vi "Inspect Tell.vi"(4 "Alias":string, 6 "Msg":refnum<class "Msg.lvclass">, 10 "Teller":T1 {"Absolute Time" format="%<%x %.3X>T"}, 11 "Base Actor in":refnum<class "Base Actor.lvclass">) -> (0 "Error out":errorcluster, 3 "Base Actor out":refnum<class "Base Actor.lvclass">)   [LabVIEW 2020, in "jettl.lvlib" / "Base jettl Actor.lvlib" / "Base Actor.lvlib" / "Base Actor.lvclass"]
uses:
  Base Actor.lvclass
  Base Actor.lvclass/Base Actor.ctl
  Relation.ctl
  jettl.lvlib
  Teller.ctl
  Msg/Msg.lvclass
  Transport/Transport.lvclass
  Actor/Actor.lvclass
  Msgs.ctl
  Unified Layer.ctl
  Actor Attributes.ctl
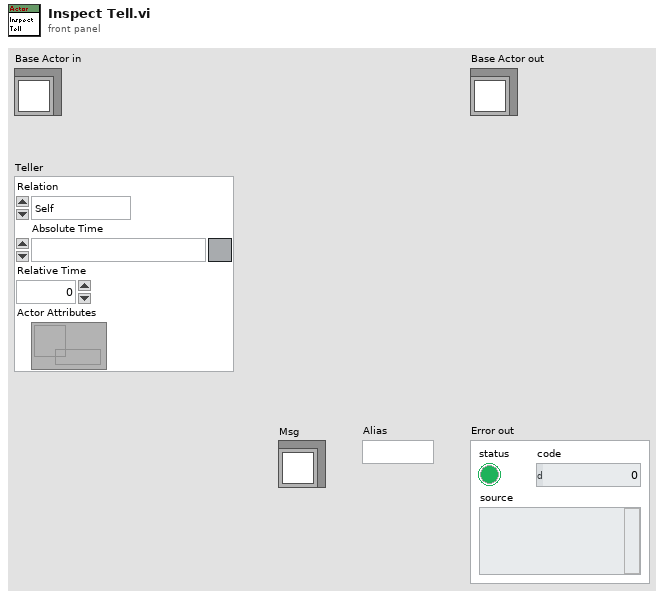
[diagram p1: front panel]
types:
  T1 = typedef "jettl.lvlib/Teller.ctl" = cluster{"Relation":T2, "Absolute Time":timestamp, "Relative Time":dbl, "Actor Attributes":refnum<data-value>}
  T2 = typedef "jettl.lvlib/Relation.ctl" = enum16{"Self", "Parent", "Child"}
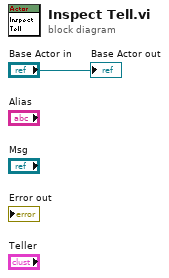
[diagram p0: block diagram]
diagram:
  "Base Actor out" <- "Base Actor in"
